vi "Close All VI References.vi"(8 "error in":errorcluster, 11 "state in":T1) -> (0 "error out":errorcluster)   [LabVIEW 2010, in "NI_SE_Config Front Panel Layout.lvlib"]
uses:
  NI_SE_Config Front Panel Layout.lvlib
  State.ctl
  VI Info.ctl
  VI Panel Layout/VI Panel Layout.lvclass
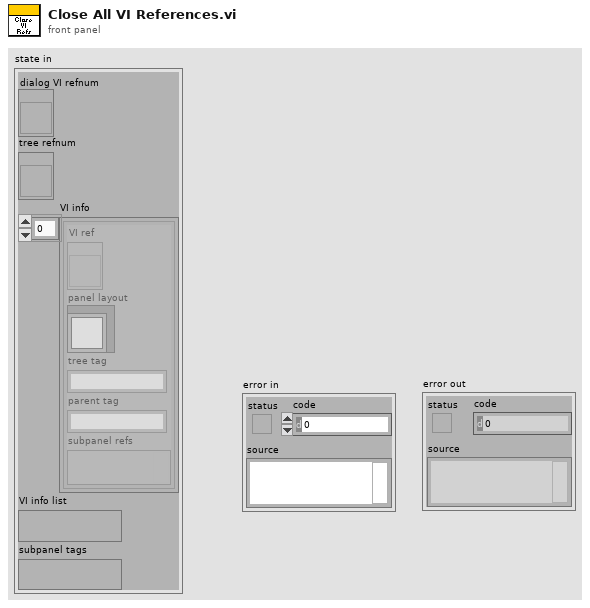
[diagram p1: front panel]
types:
  T1 = typedef "NI_SE_Config Front Panel Layout.lvlib/State.ctl" = cluster{"dialog VI refnum":refnum<vi>, "tree refnum":refnum<vi>, "VI info":T2[], "VI info list":variant, "subpanel tags":variant}
  T2 = typedef "NI_SE_Config Front Panel Layout.lvlib/VI Info.ctl" = cluster{"VI ref":refnum<vi>, "panel layout":refnum<class "VI Panel Layout.lvclass">, "tree tag":string, "parent tag":string, "subpanel refs":variant}
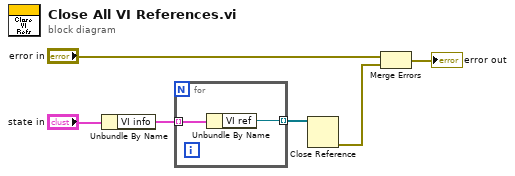
[diagram p0: block diagram]
diagram:
  n1 = Unbundle By Name("state in") -> ("VI info"=w5:T2[])
  n2 = for {
    tunnel: w5 -> [w7] mode=indexing
    tunnel: [w8] -> w1 mode=indexing
    n3 = Unbundle By Name(w7) -> ("VI ref"=w8:refnum<vi>)
  }
  n4 = Close Reference(reference=w1) -> (error out=w4:errorcluster)  [unwired: 1 in]
  n5 = Merge Errors("error in", w4) -> (→"error out":errorcluster)
